vi "LCR_FileCheck.vi"(8 "error in":errorcluster, 10 "Exists":bool, 11 "Path IN":path) -> (0 "error Out":errorcluster, 2 "Continue":bool, 3 "refnum":refnum<file>)   [LabVIEW 2021]
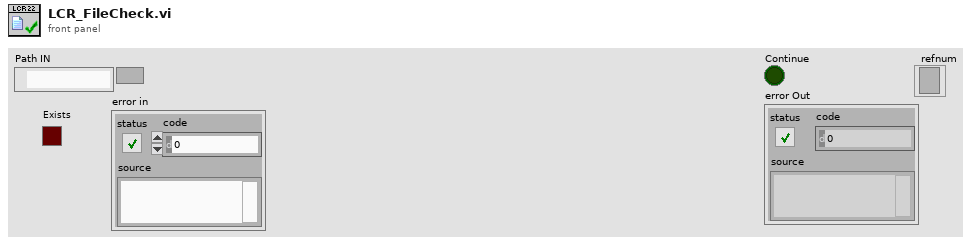
[diagram p1: front panel]
types:
  T1 = enum16{"open", "replace", "create", "open or create", "replace or create", "replace or create with confirmation"}
  T2 = enum16{"Left Button", "Center Button", "Right Button", "Window Close"}
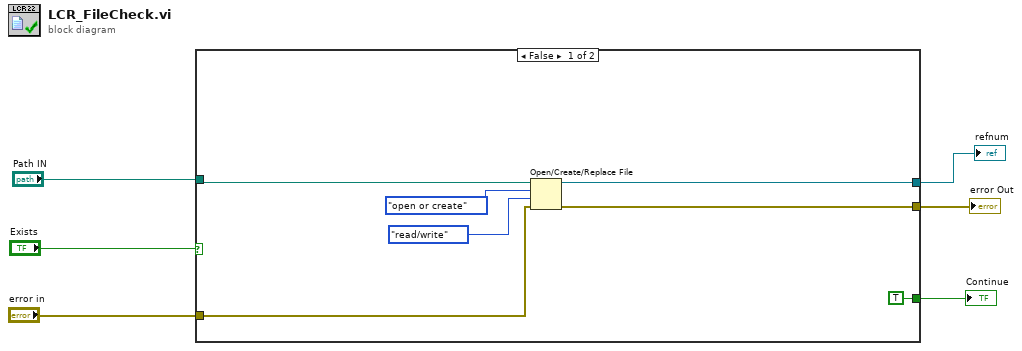
[diagram p0: block diagram]
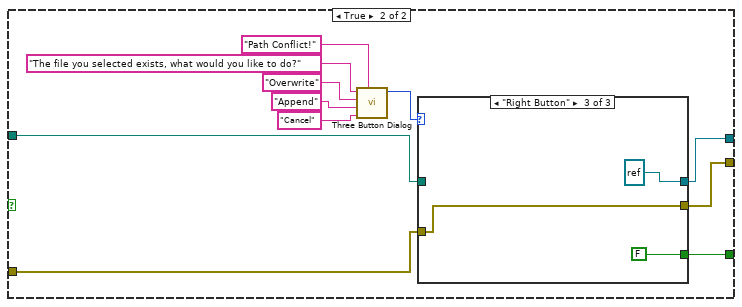
[diagram p2: hidden frame]
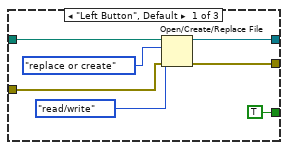
[diagram p3: hidden frame]
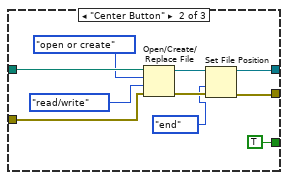
[diagram p4: hidden frame]
diagram:
  n1 = case shown="False" "Exists" {
    tunnel: "Path IN" -> [w13 w18]
    tunnel: "error in" -> [w10 w17]
    tunnel: [w9 w16] -> w1
    tunnel: [w8 w15] -> w2
    tunnel: [TRUE w14] -> w3
    frame False {
      n2 = Open/Create/Replace File(file path (use dialog)=w13, error in=w10, operation (0:open)=T1."open or create", access (0:read/write)=enum16{"read/write", "read-only", "write-only"}."read/write") -> (refnum out=w9:refnum<file>, error out=w8:errorcluster)  [unwired: 2 in, 1 out]
    }
    frame True {
      n3 = call <vilib>:"Three Button Dialog.vi"("Window Title (\"\")"="Path Conflict!" ("Window Title (\"\")"), "Right Button Text (\"Cancel\")"="Cancel" ("Right Button Text (\"Cancel\")"), "Center Button Text (\"No\")"="Append" ("Center Button Text (\"No\")"), "Left Button Text (\"Yes\")"="Overwrite" ("Left Button Text (\"Yes\")"), "message"="The file you selected exists, what would you like to do?") -> ("Which Button?"=w19:T2)  [unwired: 6 in]
      n4 = case shown="\"Right Button\"" w19 {
        tunnel: w18 -> [w31 w41 _]
        tunnel: w17 -> [w30 w40 w43]
        tunnel: [w27 w38 refnum<file> refnum ("refnum")] -> w16
        tunnel: [w26 w37 w43] -> w15
        tunnel: [TRUE TRUE FALSE] -> w14
        frame "Left Button", Default {
          n5 = Open/Create/Replace File(file path (use dialog)=w31, error in=w30, operation (0:open)=T1."replace or create", access (0:read/write)=enum16{"read/write", "read-only", "write-only"}."read/write") -> (refnum out=w27:refnum<file>, error out=w26:errorcluster)  [unwired: 2 in, 1 out]
        }
        frame "Center Button" {
          n6 = Open/Create/Replace File(file path (use dialog)=w41, error in=w40, operation (0:open)=T1."open or create", access (0:read/write)=enum16{"read/write", "read-only", "write-only"}."read/write") -> (refnum out=w39:refnum<file>, error out=w36:errorcluster)  [unwired: 2 in, 1 out]
          n7 = Set File Position(refnum=w39, from (0:start)=enum16{"start", "end", "current"}."end", error in=w36) -> (refnum out=w38:refnum<file>, error out=w37:errorcluster)  [unwired: 1 in]
        }
        frame "Right Button" {
        }
      }
    }
  }
  "Continue" <- w3
  "error Out" <- w2
  "refnum" <- w1
